vi "authorize email request.vi"(8 "error in (no error)":errorcluster, 11 "POST (empty)":T1) -> (0 "error out":errorcluster)   [LabVIEW 2011]
uses:
  Addons/internet/utils/keyedarr.llb/Keyed Array.ctl
  Addons/internet/utils/strutil.llb/Case Matching.ctl
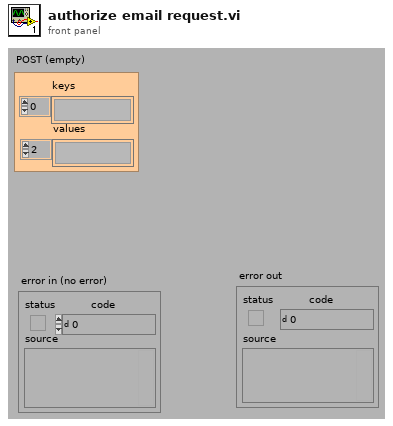
[diagram p1: front panel]
types:
  T1 = typedef "Keyed Array.ctl" = cluster{"keys":string[], "values":string[]}
  T2 = cluster{"Server":string, "Send Username":string, "Send Password":string, "Connection Timeout, s":i32}
  T3 = typedef "Case Matching.ctl" = enum16{"a != A", "a == A", "system"}
  T4 = cluster{"To (\"\")":string, "From (\"\")":string, "Subject (\"\")":string, "HTMLBody (\"\")":string}
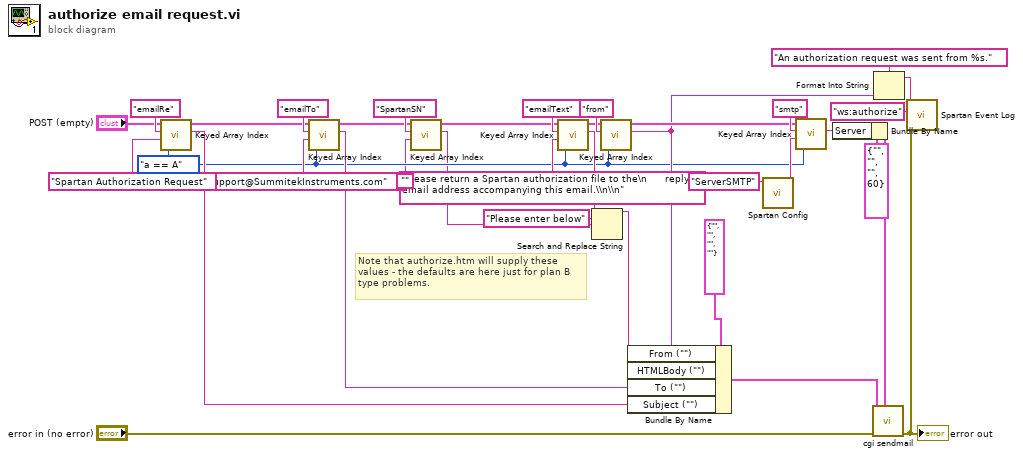
[diagram p0: block diagram]
diagram:
  w6 = Case_Matching."a == A" ("case matching (sensitive)")
  # "Note that authorize.htm will supply these\nvalues - the defaults are here just for plan B\ntype problems."
  n1 = call "Keyed Array Index.vi"("case matching (sensitive)"=w6, "default value"="Spartan Authorization Request" ("key"), "key"="emailRe", "array in"="POST (empty)") -> ("value"=w13:string, "duplicate array"=w16:T1)  [unwired: 2 out]
  n2 = call "Keyed Array Index.vi"("case matching (sensitive)"=w6, "default value"="Support@SummitekInstruments.com" ("key"), "key"="emailTo", "array in"=w16) -> ("value"=w18:string, "duplicate array"=w3:T1)  [unwired: 2 out]
  n3 = call "Keyed Array Index.vi"("default value"="" ("key"), "key"="SpartanSN", "array in"=w3) -> ("value"=w1:string, "duplicate array"=w2:T1)  [unwired: 1 in, 2 out]
  n4 = call "Keyed Array Index.vi"("case matching (sensitive)"=w6, "default value"="Please return a Spartan authorization file to the\n      reply-to email address accompanying this email.\\n\\n" ("key"), "key"="emailText", "array in"=w2) -> ("value"=w9:string, "duplicate array"=w21:T1)  [unwired: 2 out]
  n5 = Search and Replace String(input string=w9, search string="Please enter below" ("key"), replace string=w1) -> (result string=w8:string)  [unwired: 5 in, 3 out]
  n6 = call "Keyed Array Index.vi"("case matching (sensitive)"=w6, "key"="from", "array in"=w21) -> ("value"=w23:string, "duplicate array"=w32:T1)  [unwired: 1 in, 2 out]
  n7 = Bundle By Name(cluster=T4 {"To (\"\")"="", "From (\"\")"="", "Subject (\"\")"="", "HTMLBody (\"\")"=""} ("Email Details"), "From (\"\")"=w23, "HTMLBody (\"\")"=w8, "To (\"\")"=w18, "Subject (\"\")"=w13) -> (w35:T4)
  n8 = call "Spartan Config.vi"("Config Key (\"\")"="ServerSMTP") -> ("Config Value"=w10:string)  [unwired: 8 in, 2 out]
  n9 = call "Keyed Array Index.vi"("case matching (sensitive)"=w6, "default value"=w10, "key"="smtp", "array in"=w32) -> ("value"=w29:string)  [unwired: 3 out]
  n10 = Bundle By Name(cluster=T2 {"Server"="", "Send Username"="", "Send Password"="", "Connection Timeout, s"=60} ("SMTP Server Info"), "Server"=w29) -> (w30:T2)
  n11 = call "cgi sendmail.vi"("SMTP Server Info"=w30, "error in (no error)"="error in (no error)", "Email Details"=w35) -> ("error out"=w24:errorcluster)  [unwired: 1 in, 4 out]
  "error out" <- w24
  n12 = Format Into String(format string="An authorization request was sent from %s." ("message (\"\")"), w23) -> (resulting string=w27:string)  [unwired: 2 in, 1 out]
  n13 = call "Spartan Event Log.vi"("error in (no error)"=w24, "module (\"\")"="ws:authorize" ("module (\"\")"), "message (\"\")"=w27) -> ()  [unwired: 5 in, 1 out]
